vi "CloseCalcPanel.vi"(8 "error in (no error)":errorcluster caption="entrée d'erreur (pas d'erreur)", 10 "SubPanRef":refnum<vi>, 11 "PanelViRefOut":refnum<vi>[](array[refnum])) -> (0 "sortie d'erreur":errorcluster)   [LabVIEW 2019]
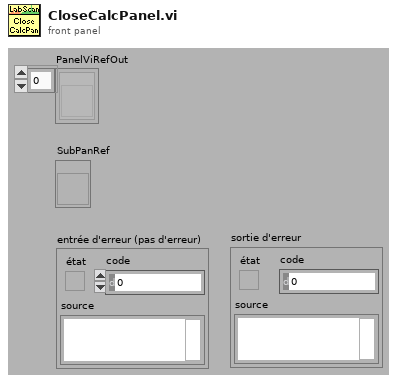
[diagram p1: front panel]
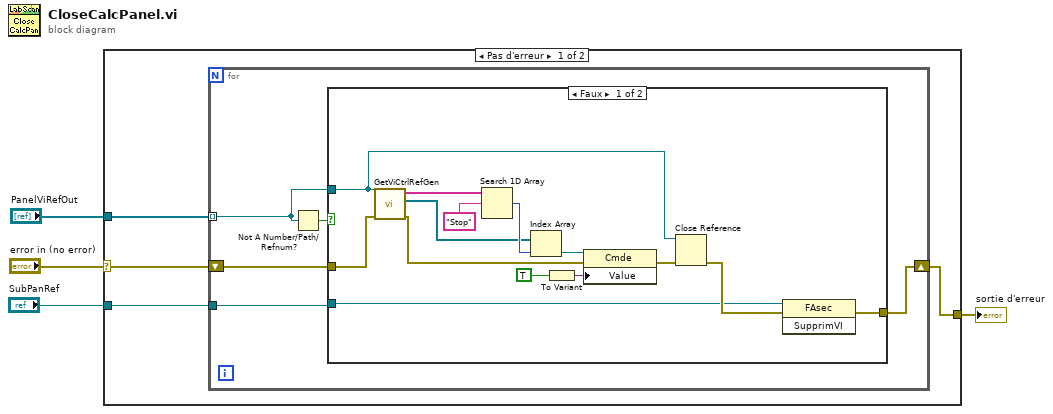
[diagram p0: block diagram]
diagram:
  n1 = case shown="Pas d'erreur" "error in (no error)" {
    selector: "error in (no error)" -> [w8 w29]
    tunnel: [w7 w29] -> w3
    tunnel: "SubPanRef" -> [w6 _]
    tunnel: "PanelViRefOut" -> [w5 _]
    frame No Error {
      n2 = for {
        tunnel: w6 -> [w11]
        tunnel: w5 -> [w9] mode=indexing
        shift-right: [w12] -> w7
        shift-left: w8 -> [w13]
        n3 = Not A Number/Path/Refnum?(number/path/refnum=w9) -> (NaN/Path/Refnum?=w10:bool)
        n4 = case shown="Faux" w10 {
          tunnel: w13 -> [w27 w28]
          tunnel: [w26 w28] -> w12
          tunnel: w9 -> [w15 _]
          tunnel: w11 -> [w14 _]
          frame False {
            n5 = call <userlib>:"GetViCtrlRefGen.vi"("ErrorIn(No Error)"=w27, "VIRef"=w15) -> ("sortie d'erreur"=w20:errorcluster, "ControlsRefs"=w23:refnum<vi>[], "ControlsNames"=w25:string[])  [unwired: 7 in]
            n6 = Search 1D Array(1D array=w25, element="Stop") -> (index of element=w24:i32)  [unwired: 1 in]
            n7 = Index Array(array=w23, index=w24) -> (element=w21:refnum<vi>)
            n8 = To Variant(anything=TRUE) -> (Variant=w18:variant)
            n9 = property class="Cmde"(reference=w21, error in=w20, "Value"=w18) -> (error out=w17:errorcluster)  [unwired: 1 out]
            n10 = Close Reference(reference=w15, error in (no error)=w17) -> (error out=w16:errorcluster)
            n11 = invoke class="FAsec" method="SupprimVI"(reference=w14, error in=w16) -> (error out=w26:errorcluster)  [unwired: 1 in, 2 out]
          }
          frame True {
          }
        }
      }
    }
    frame Error {
    }
  }
  "sortie d'erreur" <- w3
